vi "ReadHeadFast.vi"(9 "Use File?":bool=TRUE, 10 "raw reader":string, 11 "new file path":path=path "C:/WINDOWS/DESKTOP/rri.eye") -> (3 "refnum out":refnum<file>, 5 "Header In":T3={"header info"={"Header"="", "Head length"=0}, "A/D info"={"# rf points per line"=0, "# lines per scan"=0, "sample rate MHz"=0, "# A/D bits"=0, "# bytes per A/D"=0, "TGC Flag"=0, "A/D Type"=""}, "Tranducer Info"={"bandwidth"=0.0, "center freq"=0.0, "start freq"=0.0, "ID"=0}, "Scan Info"={"delay"=0.0, "pivot distance"=0.0, "sector scan angle"=0.0, "operator"="", "Scan Mode"="", "location"=""}, "Time/Date Info"={"date"="", "time"=""}, "RF Info"={"RF file name"="", "RF file att"="", "RF cal file name"="", "RF cal file att"=""}, "Patient Info"={"ID"="", "extended ID"="", "age"=0, "sex"="", "previously\nscanned"="", "PSA"=0.0, "LOS"=1, "Ethnicty 2"=3, "Race"=3}, "Tissue Type"={"organ"=0, "disease type"=0, "disease location"=0, "IQ_pts"=0, "RcvBuffer"=0, "RcvFrame"=0, "IQBuff"=0, "IQFrame"=0, "IQPage"=0}, "Votage scaling"={"Digitizer (dB)"=0.0, "Gain (dB)"=0.0, "Atten (dB)"=0.0}, "Comment"="", "Misc Info"={"avg num"=0, "c speed"=0, "Div By or SF zones"=0, "XMIT CHS"=0, "RCV CHS"=0, "Xmit angle"=0.0}, "Therapy Parameters"={"Theraputic Freq (MHz)"=0.1, "Time on (s)"=1.0, "Therapy amplitude (mV)"=50.0, "Lines Before"=20, "Lines After"=80}, "Scan Settings"={"Energy (uJ or V)"=0, "Damp (Ohm) or Fc"=0, "HP Filt (KHz)"=0, "LP Filt (MHz)"=0, "Gain (db)"=0, "prf (kHz)"=0.0, "Distance between\nscan lines (um)"=0, "Distance between\nscan planes (um)"=0, "Scan line gap (um)"=0.0, "Scan plane gap (um)"=0.0}, "Compression Parameters"={"F1 (MHz)"=0.0, "F2 (MHz)"=0.0, "% taper"=0.0, "duration"=0.0}, "Patient Info Xtra"={"First Name"="", "Last Name"="", "Notes"=""}, "ROI Box"=[]} {"Compression Parameters"."% taper" min=50 max=1000 format="%.2f"; "Compression Parameters"."F2 (MHz)" format="%.3f"; "Compression Parameters"."F1 (MHz)" format="%.3f"; "Scan Settings"."prf (kHz)" format="%.2f"; "Therapy Parameters"."Therapy amplitude (mV)" min=50 max=1000 format="%.2f"; "Therapy Parameters"."Time on (s)" format="%.3f"; "Therapy Parameters"."Theraputic Freq (MHz)" format="%.3f"; "Patient Info"."Race" items=["Am Ind or Alaska", "Asian", "Hawaiian, Pac Isl", "Black or Afr Amer", "White", "more than one race", "unknown"]; "Patient Info"."Ethnicty 2" items=["Hispanic", "Non-Hispanic", "unknown"]; "Patient Info"."LOS" items=["1", "2", "3", "4", "5"]; "Patient Info"."PSA" format="%.1f"; "Scan Info"."delay" format="%.2f"; "Scan Info"."pivot distance" format="%.2f"; "Scan Info"."sector scan angle" format="%.2f"; "Tranducer Info"."bandwidth" format="%.2f"; "Tranducer Info"."center freq" format="%.2f"; "Tranducer Info"."start freq" format="%.2f"}, 6 "Scan Settings (Pulser and Scaping)":T4 {"prf (kHz)" format="%.2f"}, 7 "raw header out":string)   [LabVIEW 2022 SP3]
uses:
  Header.ctl
panel:
  out "filler 3":string
  out "Blank":string
  out "Patient Info Old":T1={"ID"="", "Extended ID"="", "age"=0, "gender"="", "previously\nscanned"="", "PSA"=0.0, "LOS"=1, "Ethnicty 3"=3} {"Ethnicty 3" items=["Am Ind or Alaska", "Asian, Pac Islander", "Black, not Hispanic", "Hispanic", "White, not hispanic", "other, unknown"]; "LOS" items=["1", "2", "3", "4", "5"]; "PSA" format="%.1f"}
  out "blank":i16
  out "Non-5900 Scan Setting":T2={"Flag"=0, "Puls mode"=3, "Voltage [V]"=0, "Freq. [MHz]"=0, "Gain [dB]"=0, "not used"=0.0, "Distance between\nscan lines (mm)"=0, "Distance between\nscan planes (mm)"=0, "Scan line gap (um)"=0.0, "Scan plane gap (um)"=0.0} {"Puls mode" items=["Half cycle positive", "Half cycle negegative", "Full cycle positive", "Full cycle negative"]; "not used" format="%.2f"}
  out "Ethnicty":u8(ring)=3 items=["Am Ind or Alaska", "Asian, Pac Islander", "Black, not Hispanic", "Hispanic", "White, not hispanic", "other, unknown"]
  # "© 2001-2014\nRiverside Research Institute"
  # "Old style race indicator"
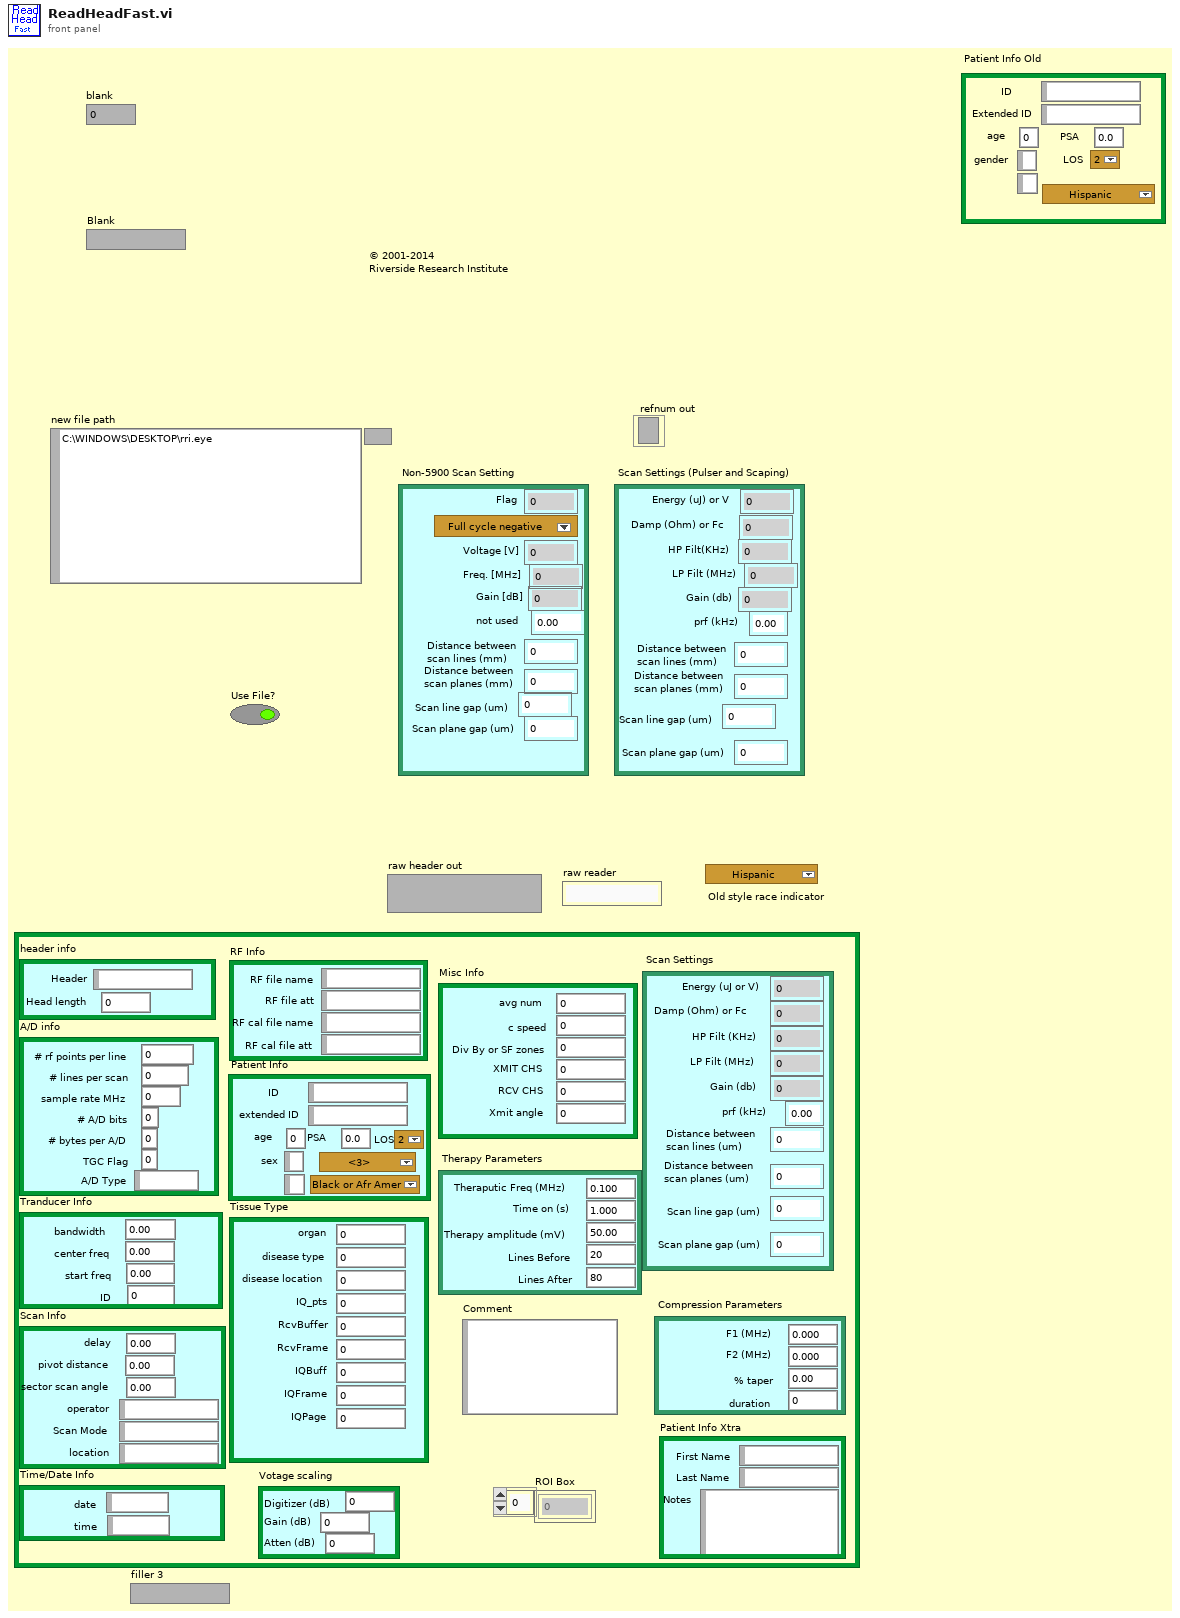
[diagram p1: front panel]
types:
  T1 = cluster{"ID":string, "Extended ID":string, "age":u16, "gender":string, "previously\nscanned":string, "PSA":sgl, "LOS":u8, "Ethnicty 3":u8}
  T2 = cluster{"Flag":u8, "Puls mode":u16, "Voltage [V]":u8, "Freq. [MHz]":u8, "Gain [dB]":u8, "not used":sgl, "Distance between\nscan lines (mm)":u16, "Distance between\nscan planes (mm)":u16, "Scan line gap (um)":sgl, "Scan plane gap (um)":sgl}
  T3 = typedef "Header.ctl" = cluster{"header info":cluster{"Header":string, "Head length":i16}, "A/D info":cluster{"# rf points per line":u16, "# lines per scan":u16, "sample rate MHz":u16, "# A/D bits":i16, "# bytes per A/D":u16, "TGC Flag":u16, "A/D Type":string}, "Tranducer Info":cluster{"bandwidth":sgl, "center freq":sgl, "start freq":sgl, "ID":i32}, "Scan Info":cluster{"delay":sgl, "pivot distance":sgl, "sector scan angle":sgl, "operator":string, "Scan Mode":string, "location":string}, "Time/Date Info":cluster{"date":string, "time":string}, "RF Info":cluster{"RF file name":string, "RF file att":string, "RF cal file name":string, "RF cal file att":string}, "Patient Info":cluster{"ID":string, "extended ID":string, "age":u16, "sex":string, "previously\nscanned":string, "PSA":sgl, "LOS":u8, "Ethnicty 2":u8, "Race":u8}, "Tissue Type":cluster{"organ":i16, "disease type":i16, "disease location":i16, "IQ_pts":u16, "RcvBuffer":u8, "RcvFrame":u16, "IQBuff":u8, "IQFrame":u16, "IQPage":u8}, "Votage scaling":cluster{"Digitizer (dB)":sgl, "Gain (dB)":sgl, "Atten (dB)":sgl}, "Comment":string, "Misc Info":cluster{"avg num":u16, "c speed":i16, "Div By or SF zones":i16, "XMIT CHS":u8, "RCV CHS":u8, "Xmit angle":sgl}, "Therapy Parameters":cluster{"Theraputic Freq (MHz)":sgl, "Time on (s)":sgl, "Therapy amplitude (mV)":sgl, "Lines Before":u16, "Lines After":u16}, "Scan Settings":cluster{"Energy (uJ or V)":u8, "Damp (Ohm) or Fc":u8, "HP Filt (KHz)":u8, "LP Filt (MHz)":u8, "Gain (db)":u8, "prf (kHz)":sgl, "Distance between\nscan lines (um)":u16, "Distance between\nscan planes (um)":u16, "Scan line gap (um)":sgl, "Scan plane gap (um)":sgl}, "Compression Parameters":cluster{"F1 (MHz)":sgl, "F2 (MHz)":sgl, "% taper":sgl, "duration":sgl}, "Patient Info Xtra":cluster{"First Name":string, "Last Name":string, "Notes":string}, "ROI Box":u16[]}
  T4 = cluster{"Energy (uJ) or V":u8, "Damp (Ohm) or Fc":u8, "HP Filt(KHz) ":u8, "LP Filt (MHz)":u8, "Gain (db)":u8, "prf (kHz)":sgl, "Distance between\nscan lines (mm)":u16, "Distance between\nscan planes (mm)":u16, "Scan line gap (um)":sgl, "Scan plane gap (um)":sgl}
  T5 = cluster{"Index":u16, "Index":u16, "Index":u16, "Index":u16, "Index":u16, "Index":u16, "raw reader":string}
  T6 = cluster{sgl, sgl, sgl, "raw reader":string, "raw reader":string, "raw reader":string}
  T7 = cluster{"raw reader":string, "raw reader":string}
  T8 = cluster{"raw reader":string, "raw reader":string, "raw reader":string, "raw reader":string}
  T9 = cluster{"raw reader":string, "raw reader":string, u16, "raw reader":string, "raw reader":string, sgl, i32, i32, i32}
  T10 = cluster{"raw reader":string, "raw reader":string, u16, "raw reader":string, "raw reader":string, sgl, i32, i32}
  T11 = cluster{"Index":i16, "Index":i16, "Index":i16, u16, "Index":u8, u16, "Index":u8, u16, "Index":u8}
  T12 = cluster{u16, "Index":i16, "Index":i16, "Index":u8, "Index":u8, sgl}
  T13 = cluster{u8, u8, u8, u8, u8, sgl, u16, u16, sgl, sgl}
  T14 = cluster{"raw reader":string, "raw reader":string, "raw reader":string}
  T15 = cluster{cluster{"raw reader":string, i16}, cluster{"Index":u16, "Index":u16, "Index":u16, "Index":u16, "Index":u16, "Index":u16, "raw reader":string}, cluster{sgl, sgl, sgl, i32}, cluster{sgl, sgl, sgl, "raw reader":string, "raw reader":string, "raw reader":string}, cluster{"raw reader":string, "raw reader":string}, cluster{"raw reader":string, "raw reader":string, "raw reader":string, "raw reader":string}, cluster{"raw reader":string, "raw reader":string, u16, "raw reader":string, "raw reader":string, sgl, i32, i32, i32}, cluster{"Index":i16, "Index":i16, "Index":i16, u16, "Index":u8, u16, "Index":u8, u16, "Index":u8}, cluster{sgl, sgl, sgl}, "raw reader":string, cluster{u16, "Index":i16, "Index":i16, "Index":u8, "Index":u8, sgl}, cluster{sgl, sgl, sgl, u16, u16}, cluster{u8, u8, u8, u8, u8, sgl, u16, u16, sgl, sgl}, cluster{sgl, sgl, sgl, sgl}, cluster{"raw reader":string, "raw reader":string, "raw reader":string}, u16[]}
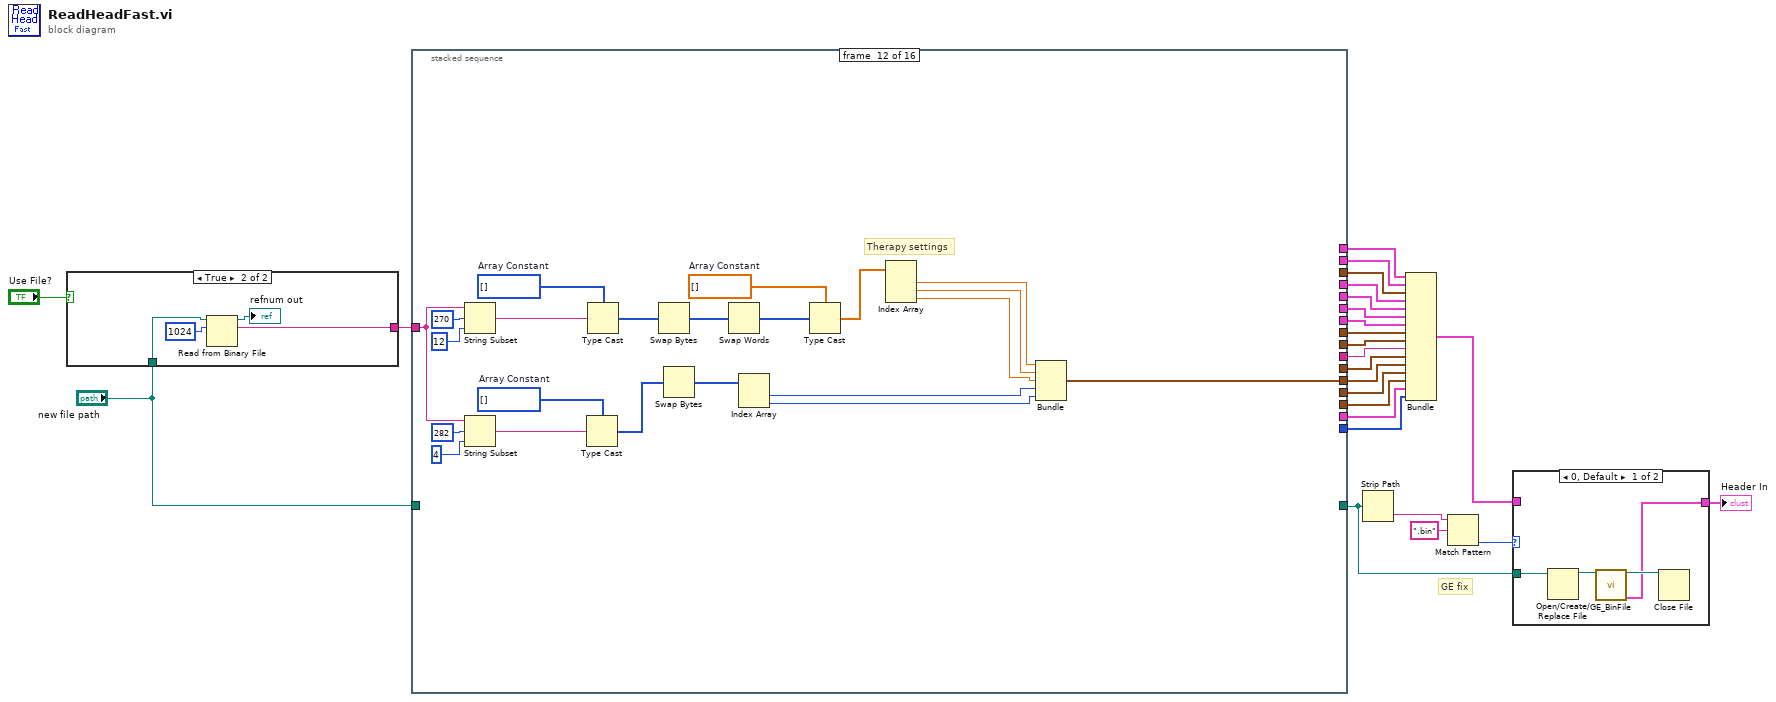
[diagram p0: block diagram]
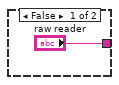
[diagram p3: hidden frame]
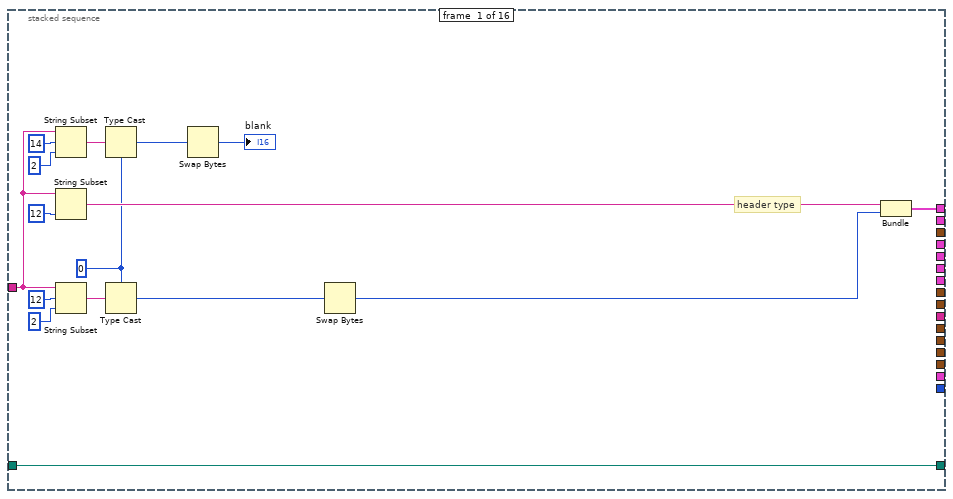
[diagram p4: hidden frame]
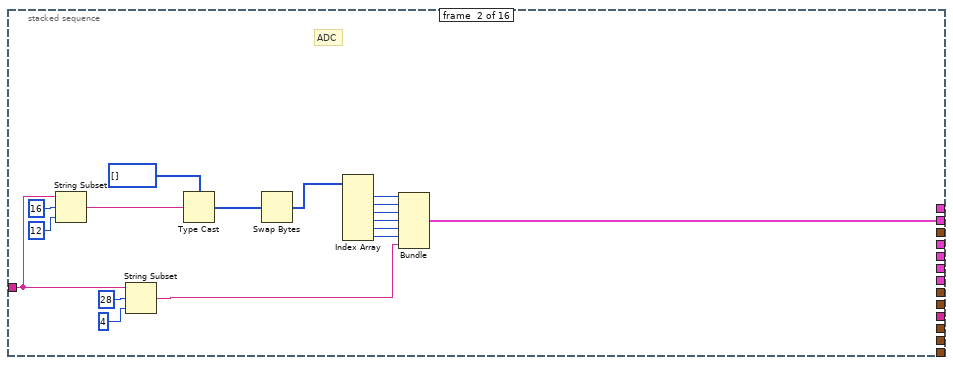
[diagram p5: hidden frame]
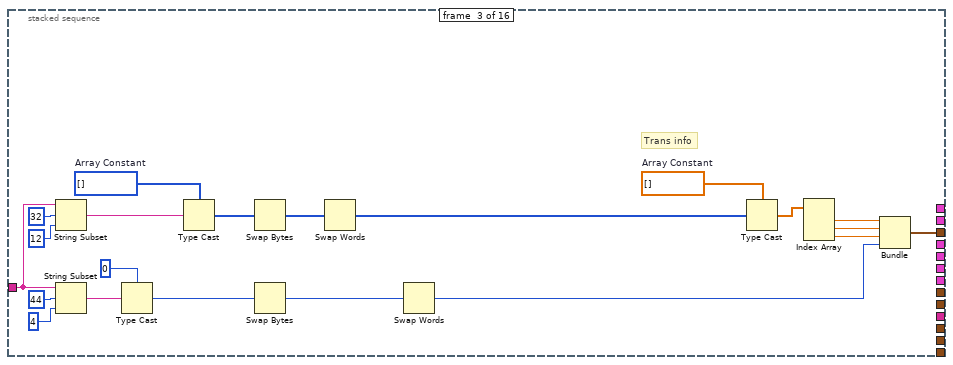
[diagram p6: hidden frame]
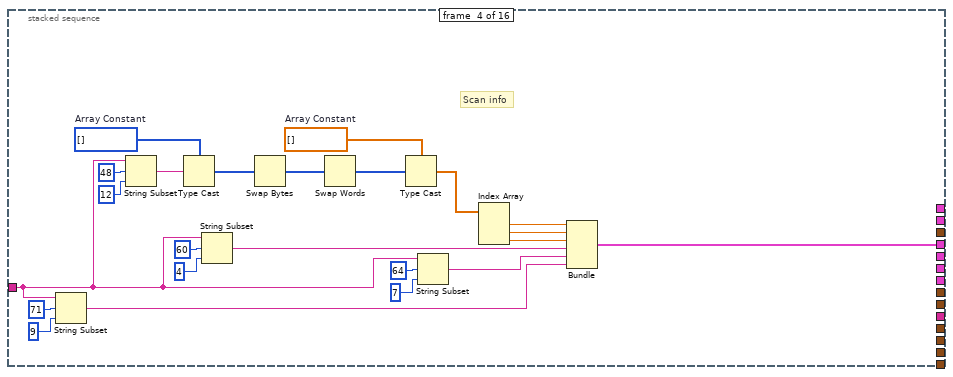
[diagram p7: hidden frame]
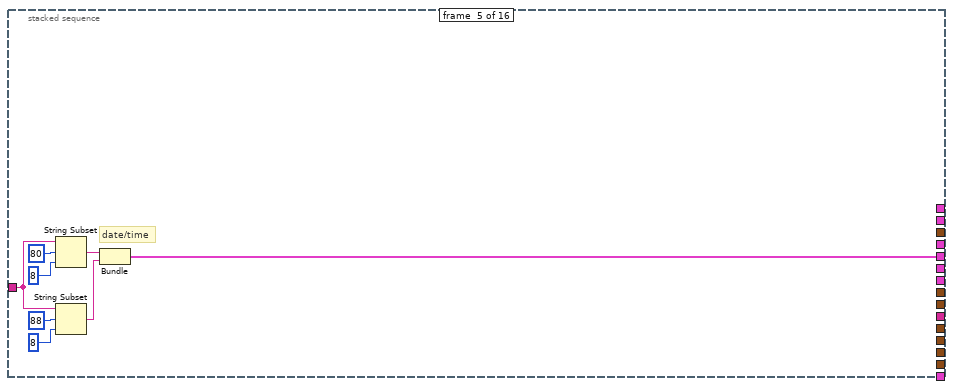
[diagram p8: hidden frame]
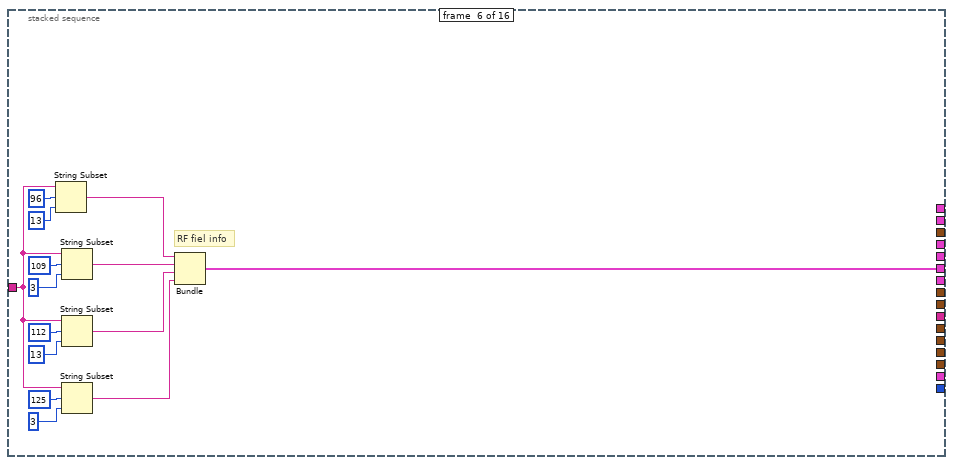
[diagram p9: hidden frame]
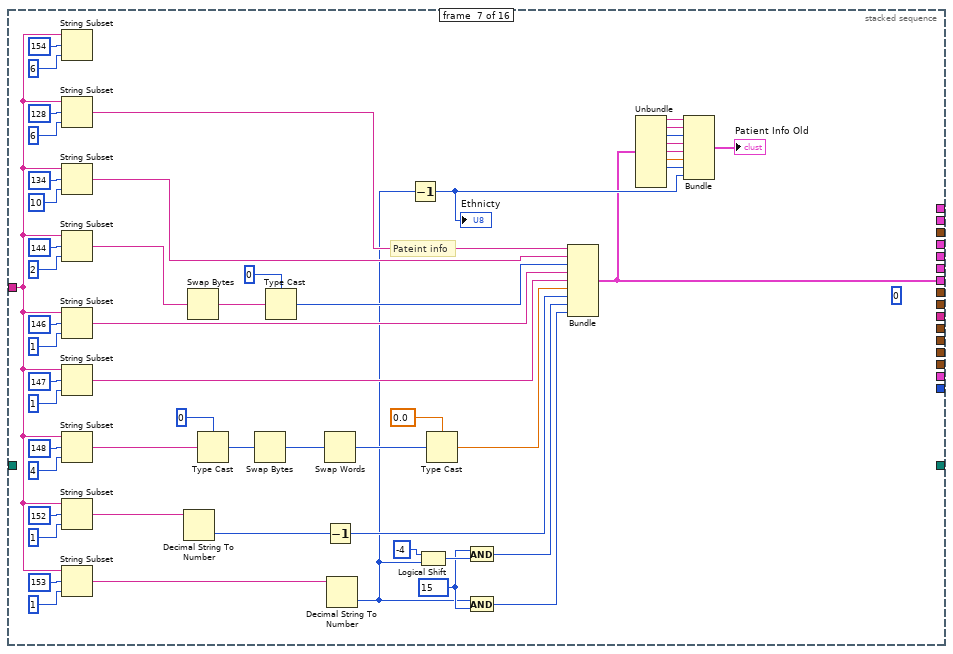
[diagram p10: hidden frame]
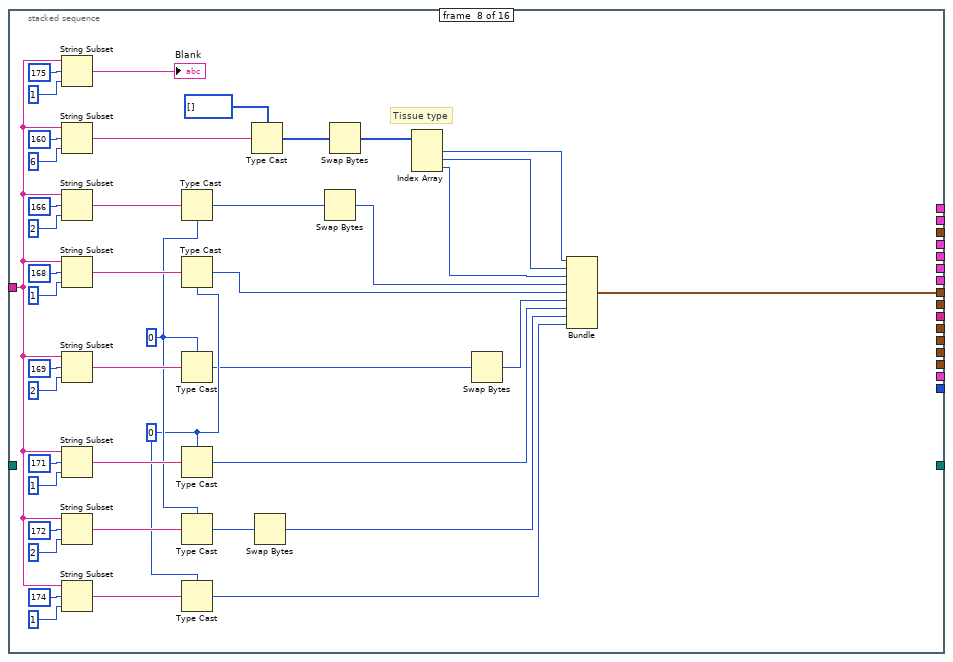
[diagram p11: hidden frame]
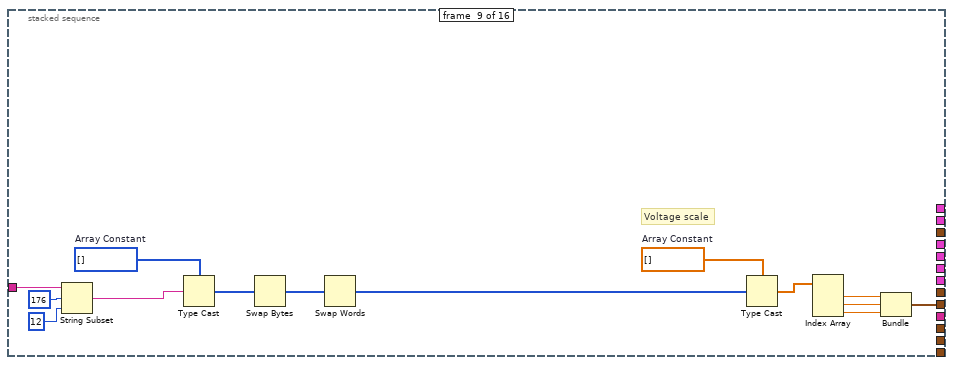
[diagram p12: hidden frame]
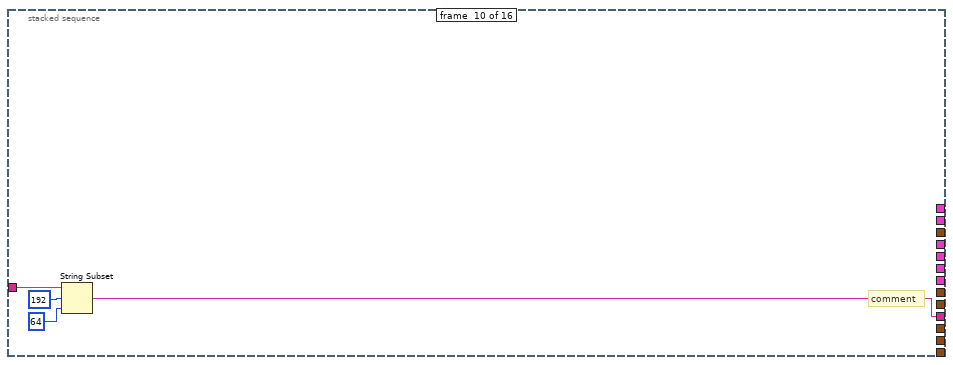
[diagram p13: hidden frame]
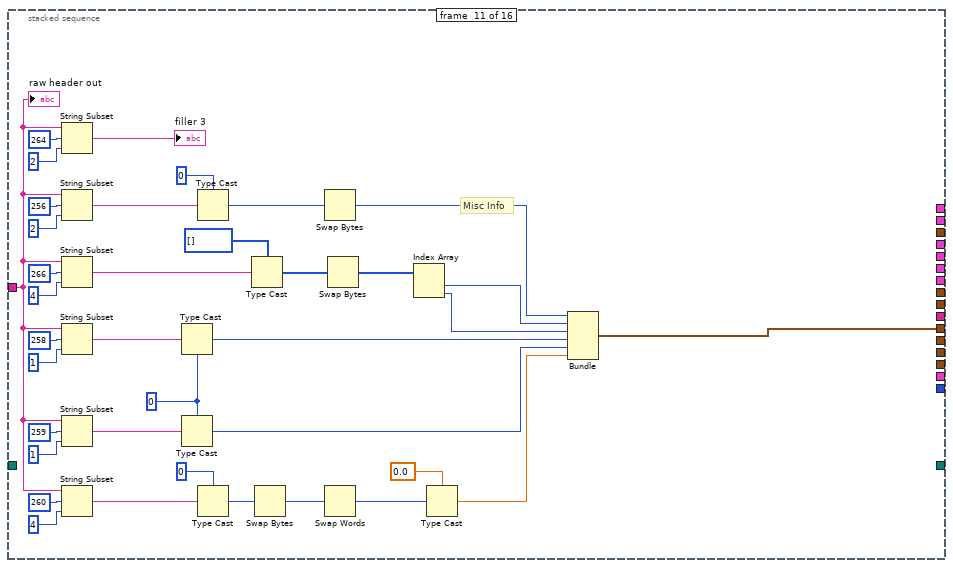
[diagram p14: hidden frame]
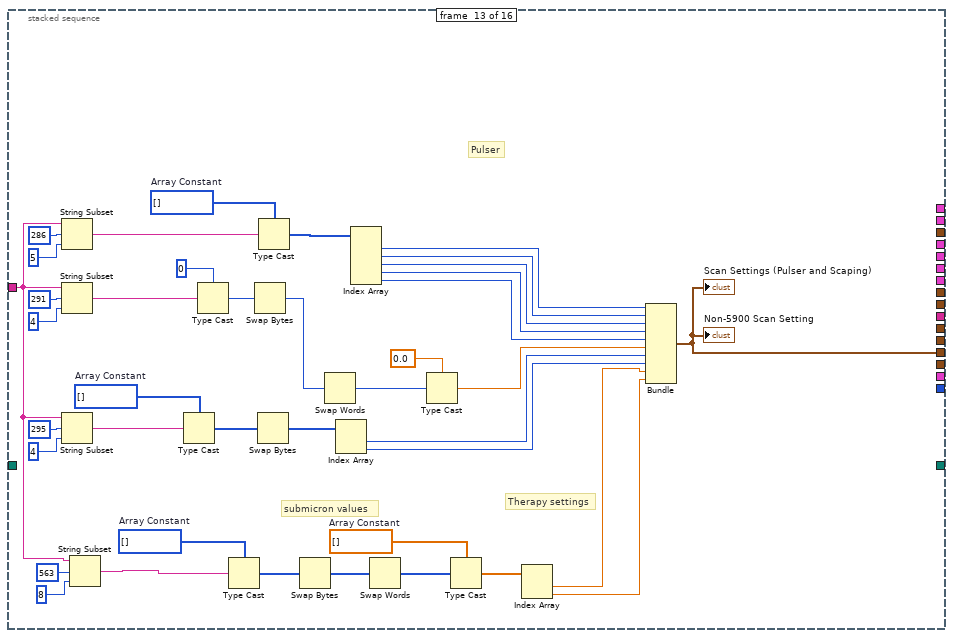
[diagram p15: hidden frame]
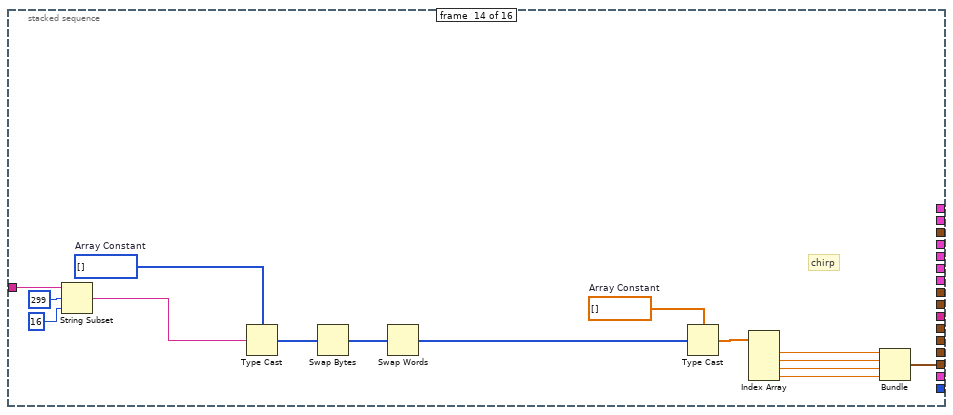
[diagram p16: hidden frame]
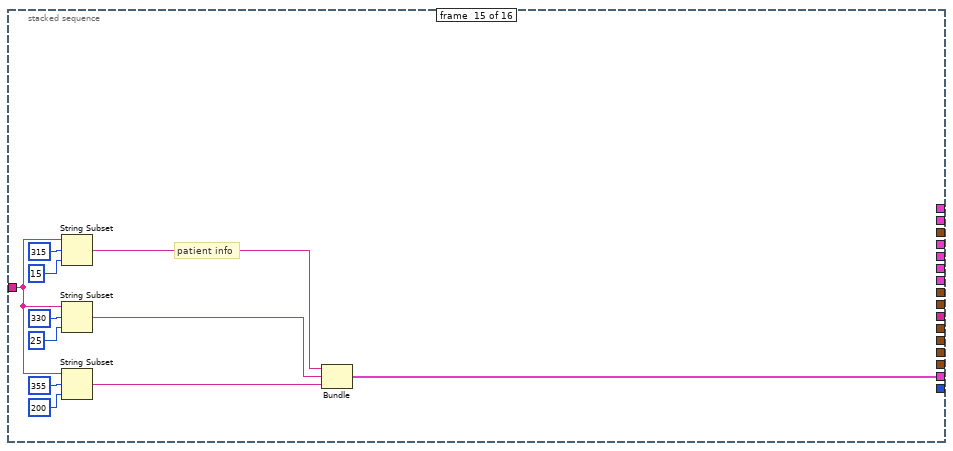
[diagram p17: hidden frame]
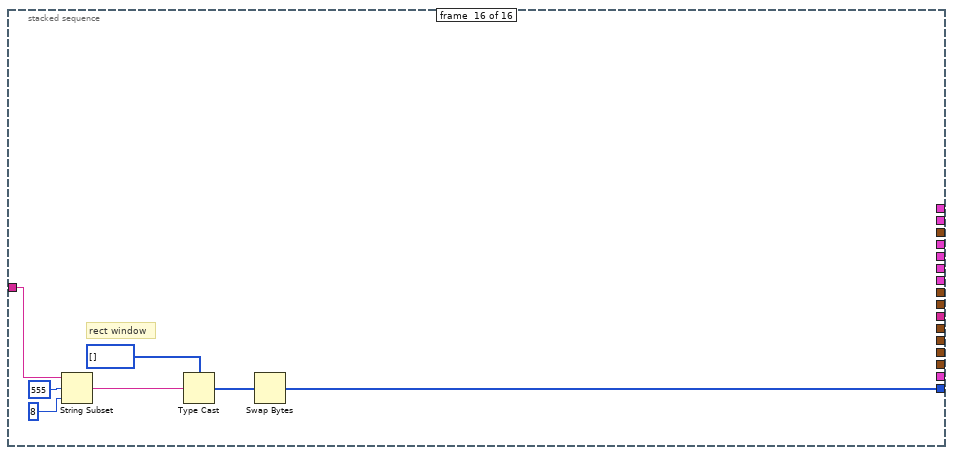
[diagram p18: hidden frame]
diagram:
  # "GE fix"
  n1 = case shown="True" "Use File?" {
    tunnel: ["raw reader" w29] -> w19
    tunnel: "new file path" -> [_ w27]
    frame False {
    }
    frame True {
      n2 = Read from Binary File(10:1024, 11:w27) -> (2:w29:string, 3:→"refnum out":refnum<file>)  [unwired: 1 in, 5 out]
    }
  }
  n3 = stacked-sequence {
    tunnel: [w41 _ _ _ _ _ _ _ _ _ _ _ _ _ _ _] -> w25
    tunnel: [_ _ _ w103 _ _ _ _ _ _ _ _ _ _ _ _] -> w24
    tunnel: [_ _ _ _ w113 _ _ _ _ _ _ _ _ _ _ _] -> w23
    tunnel: [_ _ _ _ _ _ _ _ _ w244 _ _ _ _ _ _] -> w22
    tunnel: [_ _ _ _ _ w125 _ _ _ _ _ _ _ _ _ _] -> w21
    tunnel: w19 -> [w45 w60 w82 w102 w109 w116 w164 w204 w234 w241 w247 w301 w319 w355 w360 w374]
    tunnel: [_ _ _ _ _ _ _ _ _ _ _ _ _ w357 _ _] -> w20
    tunnel: [_ w58 _ _ _ _ _ _ _ _ _ _ _ _ _ _] -> w18
    tunnel: [_ _ w80 _ _ _ _ _ _ _ _ _ _ _ _ _] -> w17
    tunnel: [_ _ _ _ _ _ w138 _ _ _ _ _ _ _ _ _] -> w16
    tunnel: [_ _ _ _ _ _ _ w220 _ _ _ _ _ _ _ _] -> w15
    tunnel: [_ _ _ _ _ _ _ _ w229 _ _ _ _ _ _ _] -> w14
    tunnel: [_ _ _ _ _ _ _ _ _ _ w279 _ _ _ _ _] -> w13
    tunnel: [_ _ _ _ _ _ _ _ _ _ _ w295 _ _ _ _] -> w12
    tunnel: [_ _ _ _ _ _ _ _ _ _ _ _ w331 _ _ _] -> w11
    tunnel: [_ _ _ _ _ _ _ _ _ _ _ _ _ _ w359 _] -> w9
    tunnel: [_ _ _ _ _ _ _ _ _ _ _ _ _ _ _ w370] -> w8
    tunnel: [w31 _ _ _ _ _ _ _ _ _ _ _ _ _ _ _] -> w3
    tunnel: "new file path" -> [w31 _ _ _ _ _ _ _ _ _ _ _ _ _ _ _]
    frame #0 {
      w42 = i16 0 ("Index")
      # "header type"
      n4 = String Subset(string=w45, offset (0)=14 ("count"), length (rest)=2) -> (substring=w34:string)
      n5 = String Subset(string=w45, length (rest)=12 ("count")) -> (substring=w46:string)  [unwired: 1 out]
      n6 = String Subset(string=w45, offset (0)=12 ("count"), length (rest)=2) -> (substring=w37:string)
      n7 = Type Cast(type=w42, x=w34) -> (*(type *) &x=w33:i16)
      n8 = Type Cast(type=w42, x=w37) -> (*(type *) &x=w36:i16)
      n9 = Swap Bytes(anything=w33) -> (byte swapped=→"blank":i16)
      n10 = Swap Bytes(anything=w36) -> (byte swapped=w35:i16)
      n11 = Bundle("raw reader"=w46, w35) -> (w41:cluster{"raw reader":string, i16})  [unwired: 1 out]
    }
    frame #1 {
      # "ADC"
      n12 = String Subset(string=w60, offset (0)=16 ("pos offset (0)"), length (rest)=12 ("count")) -> (substring=w54:string)
      n13 = String Subset(string=w60, offset (0)=28, length (rest)=4 ("count")) -> (substring=w62:string)
      n14 = Type Cast(type=u16[] [], x=w54) -> (*(type *) &x=w53:u16[])
      n15 = Swap Bytes(anything=w53) -> (byte swapped=w52:u16[])
      n16 = Index Array(array=w52) -> (element #1=w63:u16, element #2=w51:u16, element #3=w50:u16, element #4=w49:u16, element #5=w48:u16, element #6=w47:u16)  [unwired: 6 in]
      n17 = Bundle("Index"=w63, "Index"=w51, "Index"=w50, "Index"=w49, "Index"=w48, "Index"=w47, "raw reader"=w62) -> (w58:T5)  [unwired: 1 out]
    }
    frame #2 {
      w68 = sgl[] []  # Array Constant
      w84 = i32[] []  # Array Constant
      # "Trans info"
      n18 = String Subset(string=w82, offset (0)=32 ("pos offset (0)"), length (rest)=12 ("count")) -> (substring=w75:string)
      n19 = String Subset(string=w82, offset (0)=44 ("count"), length (rest)=4 ("byte stream type")) -> (substring=w69:string)
      n20 = Type Cast(type=0, x=w69) -> (*(type *) &x=w70:i32)
      n21 = Type Cast(type=w84, x=w75) -> (*(type *) &x=w73:i32[])
      n22 = Swap Bytes(anything=w73) -> (byte swapped=w74:i32[])
      n23 = Swap Bytes(anything=w70) -> (byte swapped=w72:i32)
      n24 = Swap Words(1:w74) -> (0:w67:i32[])
      n25 = Swap Words(1:w72) -> (0:w71:i32)
      n26 = Type Cast(type=w68, x=w67) -> (*(type *) &x=w66:sgl[])
      n27 = Index Array(array=w66) -> (element #1=w83:sgl, element #2=w65:sgl, element #3=w64:sgl)  [unwired: 3 in]
      n28 = Bundle(w83, w65, w64, w71) -> (w80:cluster{sgl, sgl, sgl, i32})  [unwired: 1 out]
    }
    frame #3 {
      w87 = i32[] []  # Array Constant
      w88 = sgl[] []  # Array Constant
      # "Scan info"
      n29 = String Subset(string=w102, offset (0)=71 ("pos offset (0)"), length (rest)=9 ("count")) -> (substring=w104:string)
      n30 = String Subset(string=w102, offset (0)=48 ("pos offset (0)"), length (rest)=12 ("count")) -> (substring=w94:string)
      n31 = Type Cast(type=w87, x=w94) -> (*(type *) &x=w92:i32[])
      n32 = String Subset(string=w102, offset (0)=60 ("pos offset (0)"), length (rest)=4 ("count")) -> (substring=w106:string)
      n33 = Swap Bytes(anything=w92) -> (byte swapped=w93:i32[])
      n34 = Swap Words(1:w93) -> (0:w90:i32[])
      n35 = Type Cast(type=w88, x=w90) -> (*(type *) &x=w89:sgl[])
      n36 = String Subset(string=w102, offset (0)=64 ("pos offset (0)"), length (rest)=7 ("count")) -> (substring=w105:string)
      n37 = Index Array(array=w89) -> (element #1=w107:sgl, element #2=w86:sgl, element #3=w85:sgl)  [unwired: 3 in]
      n38 = Bundle(w107, w86, w85, "raw reader"=w106, "raw reader"=w105, "raw reader"=w104) -> (w103:T6)  [unwired: 1 out]
    }
    frame #4 {
      # "date/time"
      n39 = String Subset(string=w109, offset (0)=80 ("pos offset (0)"), length (rest)=8 ("count")) -> (substring=w115:string)
      n40 = String Subset(string=w109, offset (0)=88, length (rest)=8 ("count")) -> (substring=w114:string)
      n41 = Bundle("raw reader"=w115, "raw reader"=w114) -> (w113:T7)  [unwired: 1 out]
    }
    frame #5 {
      # "RF fiel info"
      n42 = String Subset(string=w116, offset (0)=96 ("pos offset (0)"), length (rest)=13 ("count")) -> (substring=w129:string)
      n43 = String Subset(string=w116, offset (0)=109, length (rest)=3 ("count")) -> (substring=w128:string)
      n44 = String Subset(string=w116, offset (0)=112, length (rest)=13 ("count")) -> (substring=w127:string)
      n45 = String Subset(string=w116, offset (0)=125, length (rest)=3 ("count")) -> (substring=w126:string)
      n46 = Bundle("raw reader"=w129, "raw reader"=w128, "raw reader"=w127, "raw reader"=w126) -> (w125:T8)  [unwired: 1 out]
    }
    frame #6 {
      w175 = 15
      (unwired) u16 0
      # "Pateint info"
      n47 = String Subset(string=w164, offset (0)=154, length (rest)=6 ("count")) -> ()  [unwired: 1 out]
      n48 = String Subset(string=w164, offset (0)=128 ("pos offset (0)"), length (rest)=6 ("count")) -> (substring=w182:string)
      n49 = String Subset(string=w164, offset (0)=134, length (rest)=10 ("count")) -> (substring=w181:string)
      n50 = String Subset(string=w164, offset (0)=144, length (rest)=2 ("count")) -> (substring=w183:string)
      n51 = String Subset(string=w164, offset (0)=146, length (rest)=1 ("count")) -> (substring=w180:string)
      n52 = String Subset(string=w164, offset (0)=147, length (rest)=1 ("count")) -> (substring=w179:string)
      n53 = String Subset(string=w164, offset (0)=148, length (rest)=4 ("count")) -> (substring=w134:string)
      n54 = String Subset(string=w164, offset (0)=152, length (rest)=1 ("count")) -> (substring=w141:string)
      n55 = String Subset(string=w164, offset (0)=153, length (rest)=1 ("count")) -> (substring=w139:string)
      n56 = Decimal String To Number(string=w141) -> (number=w140:i32)  [unwired: 3 out]
      n57 = Swap Bytes(anything=w183) -> (byte swapped=w145:string)
      n58 = Type Cast(type=0, x=w134) -> (*(type *) &x=w136:i32)
      n59 = Swap Bytes(anything=w136) -> (byte swapped=w135:i32)
      n60 = Type Cast(type=u16 0, x=w145) -> (*(type *) &x=w144:u16)
      n61 = Swap Words(1:w135) -> (0:w137:i32)
      n62 = Decrement(x=w140) -> (x-1=w178:i32)
      n63 = Decimal String To Number(string=w139) -> (number=w130:i32)  [unwired: 3 out]
      n64 = Decrement(x=w130) -> (x-1=w165:i32)
      "Ethnicty" <- w165
      n65 = Logical Shift(y=-4, x=w130) -> (x << y=w176:i32)
      n66 = Type Cast(type=sgl 0.0, x=w137) -> (*(type *) &x=w133:sgl)
      n67 = And(x=w175, y=w176) -> (x .and. y?=w174:i32)
      n68 = And(x=w130, y=w175) -> (x .and. y?=w173:i32)
      n69 = Bundle("raw reader"=w182, "raw reader"=w181, w144, "raw reader"=w180, "raw reader"=w179, w133, w178, w174, w173) -> (w138:T9)  [unwired: 1 out]
      n70 = Unbundle(w138) -> ("raw reader"=w172:string, "raw reader"=w171:string, w170:u16, "raw reader"=w169:string, "raw reader"=w168:string, w167:sgl, w166:i32)  [unwired: 2 out]
      n71 = Bundle("raw reader"=w172, "raw reader"=w171, w170, "raw reader"=w169, "raw reader"=w168, w167, w166, w165) -> (→"Patient Info Old":T10)  [unwired: 1 out]
    }
    frame #7 {
      w196 = u8 0 ("Index")
      w197 = u16 0 ("Index")
      # "Tissue type"
      n72 = String Subset(string=w204, offset (0)=175, length (rest)=1 ("count")) -> (substring=→"Blank":string)
      n73 = String Subset(string=w204, offset (0)=160 ("pos offset (0)"), length (rest)=6 ("count")) -> (substring=w217:string)
      n74 = String Subset(string=w204, offset (0)=166 ("pos offset (0)"), length (rest)=2 ("count")) -> (substring=w203:string)
      n75 = String Subset(string=w204, offset (0)=168 ("pos offset (0)"), length (rest)=1 ("count")) -> (substring=w202:string)
      n76 = String Subset(string=w204, offset (0)=169 ("pos offset (0)"), length (rest)=2 ("count")) -> (substring=w201:string)
      n77 = String Subset(string=w204, offset (0)=171 ("pos offset (0)"), length (rest)=1 ("count")) -> (substring=w198:string)
      n78 = String Subset(string=w204, offset (0)=172 ("pos offset (0)"), length (rest)=2 ("count")) -> (substring=w200:string)
      n79 = String Subset(string=w204, offset (0)=174 ("pos offset (0)"), length (rest)=1 ("count")) -> (substring=w199:string)
      n80 = Type Cast(type=w197, x=w203) -> (*(type *) &x=w187:u16)
      n81 = Type Cast(type=w196, x=w202) -> (*(type *) &x=w195:u8)
      n82 = Type Cast(type=w197, x=w201) -> (*(type *) &x=w189:u16)
      n83 = Type Cast(type=w196, x=w198) -> (*(type *) &x=w194:u8)
      n84 = Type Cast(type=w197, x=w200) -> (*(type *) &x=w191:u16)
      n85 = Type Cast(type=w196, x=w199) -> (*(type *) &x=w193:u8)
      n86 = Type Cast(type=i16[] [], x=w217) -> (*(type *) &x=w219:i16[])
      n87 = Swap Bytes(anything=w191) -> (byte swapped=w190:u16)
      n88 = Swap Bytes(anything=w187) -> (byte swapped=w186:u16)
      n89 = Swap Bytes(anything=w219) -> (byte swapped=w218:i16[])
      n90 = Index Array(array=w218) -> (element #1=w226:i16, element #2=w185:i16, element #3=w184:i16)  [unwired: 3 in]
      n91 = Swap Bytes(anything=w189) -> (byte swapped=w188:u16)
      n92 = Bundle("Index"=w226, "Index"=w185, "Index"=w184, w186, "Index"=w195, w188, "Index"=w194, w190, "Index"=w193) -> (w220:T11)  [unwired: 1 out]
    }
    frame #8 {
      w236 = i32[] []  # Array Constant
      w237 = sgl[] []  # Array Constant
      # "Voltage scale"
      n93 = String Subset(string=w234, offset (0)=176 ("pos offset (0)"), length (rest)=12 ("pos offset (0)")) -> (substring=w235:string)
      n94 = Type Cast(type=w236, x=w235) -> (*(type *) &x=w239:i32[])
      n95 = Swap Bytes(anything=w239) -> (byte swapped=w240:i32[])
      n96 = Swap Words(1:w240) -> (0:w238:i32[])
      n97 = Type Cast(type=w237, x=w238) -> (*(type *) &x=w231:sgl[])
      n98 = Index Array(array=w231) -> (element #1=w230:sgl, element #2=w227:sgl, element #3=w228:sgl)  [unwired: 3 in]
      n99 = Bundle(w230, w227, w228) -> (w229:cluster{sgl, sgl, sgl})  [unwired: 1 out]
    }
    frame #9 {
      # "comment"
      n100 = String Subset(string=w241, offset (0)=192 ("pos offset (0)"), length (rest)=64 ("count")) -> (substring=w244:string)
    }
    frame #10 {
      w260 = u8 0 ("Index")
      # "Misc Info"
      n101 = String Subset(string=w247, offset (0)=264, length (rest)=2 ("count")) -> (substring=→"filler 3":string)
      n102 = String Subset(string=w247, offset (0)=256 ("pos offset (0)"), length (rest)=2 ("count")) -> (substring=w271:string)
      n103 = String Subset(string=w247, offset (0)=266, length (rest)=4 ("count")) -> (substring=w269:string)
      n104 = String Subset(string=w247, offset (0)=258 ("pos offset (0)"), length (rest)=1 ("count")) -> (substring=w264:string)
      n105 = String Subset(string=w247, offset (0)=259 ("pos offset (0)"), length (rest)=1 ("count")) -> (substring=w261:string)
      n106 = String Subset(string=w247, offset (0)=260, length (rest)=4 ("count")) -> (substring=w250:string)
      n107 = Type Cast(type=w260, x=w264) -> (*(type *) &x=w258:u8)
      n108 = Type Cast(type=w260, x=w261) -> (*(type *) &x=w257:u8)
      n109 = Type Cast(type=u16 0 ("Index"), x=w271) -> (*(type *) &x=w270:u16)
      n110 = Type Cast(type=0, x=w250) -> (*(type *) &x=w254:i32)
      n111 = Type Cast(type=i16[] [], x=w269) -> (*(type *) &x=w268:i16[])
      n112 = Swap Bytes(anything=w254) -> (byte swapped=w253:i32)
      n113 = Swap Bytes(anything=w270) -> (byte swapped=w259:u16)
      n114 = Swap Words(1:w253) -> (0:w255:i32)
      n115 = Swap Bytes(anything=w268) -> (byte swapped=w267:i16[])
      n116 = Index Array(array=w267) -> (element #1=w281:i16, element #2=w245:i16)  [unwired: 2 in]
      n117 = Type Cast(type=sgl 0.0, x=w255) -> (*(type *) &x=w246:sgl)
      n118 = Bundle(w259, "Index"=w281, "Index"=w245, "Index"=w258, "Index"=w257, w246) -> (w279:T12)  [unwired: 1 out]
      "raw header out" <- w247
    }
    frame #11 {
      w287 = i32[] []  # Array Constant
      w288 = sgl[] []  # Array Constant
      w296 = u16[] []  # Array Constant
      # "Therapy settings"
      n119 = String Subset(string=w301, offset (0)=270 ("pos offset (0)"), length (rest)=12 ("count")) -> (substring=w286:string)
      n120 = String Subset(string=w301, offset (0)=282 ("count"), length (rest)=4) -> (substring=w292:string)
      n121 = Type Cast(type=w296, x=w292) -> (*(type *) &x=w294:u16[])
      n122 = Type Cast(type=w287, x=w286) -> (*(type *) &x=w290:i32[])
      n123 = Swap Bytes(anything=w290) -> (byte swapped=w291:i32[])
      n124 = Swap Bytes(anything=w294) -> (byte swapped=w293:u16[])
      n125 = Swap Words(1:w291) -> (0:w289:i32[])
      n126 = Index Array(array=w293) -> (element #1=w302:u16, element #2=w282:u16)  [unwired: 2 in]
      n127 = Type Cast(type=w288, x=w289) -> (*(type *) &x=w285:sgl[])
      n128 = Index Array(array=w285) -> (element #1=w303:sgl, element #2=w284:sgl, element #3=w283:sgl)  [unwired: 3 in]
      n129 = Bundle(w303, w284, w283, w302, w282) -> (w295:cluster{sgl, sgl, sgl, u16, u16})  [unwired: 1 out]
    }
    frame #12 {
      w314 = i32[] []  # Array Constant
      w315 = sgl[] []  # Array Constant
      w333 = u16[] []  # Array Constant
      w339 = u8[] []  # Array Constant
      # "submicron values"
      # "Therapy settings"
      # "Pulser"
      n130 = String Subset(string=w319, offset (0)=286 ("pos offset (0)"), length (rest)=5 ("count")) -> (substring=w341:string)
      n131 = String Subset(string=w319, offset (0)=291, length (rest)=4 ("count")) -> (substring=w322:string)
      n132 = String Subset(string=w319, offset (0)=295, length (rest)=4 ("count")) -> (substring=w330:string)
      n133 = String Subset(string=w319, offset (0)=563, length (rest)=8 ("count")) -> (substring=w312:string)
      n134 = Type Cast(type=w333, x=w330) -> (*(type *) &x=w329:u16[])
      n135 = Type Cast(type=0, x=w322) -> (*(type *) &x=w326:i32)
      n136 = Type Cast(type=w314, x=w312) -> (*(type *) &x=w317:i32[])
      n137 = Swap Bytes(anything=w326) -> (byte swapped=w327:i32)
      n138 = Swap Bytes(anything=w329) -> (byte swapped=w328:u16[])
      n139 = Type Cast(type=w339, x=w341) -> (*(type *) &x=w340:u8[])
      n140 = Swap Bytes(anything=w317) -> (byte swapped=w318:i32[])
      n141 = Swap Words(1:w327) -> (0:w325:i32)
      n142 = Index Array(array=w328) -> (element #1=w343:u16, element #2=w304:u16)  [unwired: 2 in]
      n143 = Index Array(array=w340) -> (element #1=w332:u8, element #2=w308:u8, element #3=w307:u8, element #4=w306:u8, element #5=w305:u8)  [unwired: 5 in]
      n144 = Swap Words(1:w318) -> (0:w316:i32[])
      n145 = Type Cast(type=sgl 0.0, x=w325) -> (*(type *) &x=w324:sgl)
      n146 = Type Cast(type=w315, x=w316) -> (*(type *) &x=w313:sgl[])
      n147 = Index Array(array=w313) -> (element #1=w310:sgl, element #2=w309:sgl)  [unwired: 2 in]
      n148 = Bundle(w332, w308, w307, w306, w305, w324, w343, w304, w310, w309) -> (w331:T13)  [unwired: 1 out]
      "Scan Settings (Pulser and Scaping)" <- w331
      "Non-5900 Scan Setting" <- w331
    }
    frame #13 {
      w349 = i32[] []  # Array Constant
      w350 = sgl[] []  # Array Constant
      # "chirp"
      n149 = String Subset(string=w355, offset (0)=299 ("pos offset (0)"), length (rest)=16 ("count")) -> (substring=w348:string)
      n150 = Type Cast(type=w349, x=w348) -> (*(type *) &x=w352:i32[])
      n151 = Swap Bytes(anything=w352) -> (byte swapped=w353:i32[])
      n152 = Swap Words(1:w353) -> (0:w351:i32[])
      n153 = Type Cast(type=w350, x=w351) -> (*(type *) &x=w347:sgl[])
      n154 = Index Array(array=w347) -> (element #1=w358:sgl, element #2=w346:sgl, element #3=w345:sgl, element #4=w344:sgl)  [unwired: 4 in]
      n155 = Bundle(w358, w346, w345, w344) -> (w357:cluster{sgl, sgl, sgl, sgl})  [unwired: 1 out]
    }
    frame #14 {
      # "patient info"
      n156 = String Subset(string=w360, offset (0)=315 ("pos offset (0)"), length (rest)=15 ("count")) -> (substring=w363:string)
      n157 = String Subset(string=w360, offset (0)=330 ("pos offset (0)"), length (rest)=25 ("count")) -> (substring=w362:string)
      n158 = String Subset(string=w360, offset (0)=355 ("pos offset (0)"), length (rest)=200 ("count")) -> (substring=w361:string)
      n159 = Bundle("raw reader"=w363, "raw reader"=w362, "raw reader"=w361) -> (w359:T14)  [unwired: 1 in]
    }
    frame #15 {
      # "rect window"
      n160 = String Subset(string=w374, offset (0)=555 ("pos offset (0)"), length (rest)=8 ("count")) -> (substring=w373:string)
      n161 = Type Cast(type=u16[] [], x=w373) -> (*(type *) &x=w371:u16[])
      n162 = Swap Bytes(anything=w371) -> (byte swapped=w370:u16[])
    }
  }
  n163 = Strip Path(path=w3) -> (name=w6:string)  [unwired: 1 out]
  n164 = Bundle(w25, w18, w17, w24, w23, w21, w16, w15, w14, "raw reader"=w22, w13, w12, w11, w20, w9, w8) -> (w4:T15)  [unwired: 1 out]
  n165 = Match Pattern(string=w6, regular expression=".bin") -> (offset past match=w5:i32)  [unwired: 1 in, 3 out]
  n166 = case shown="0, Default" w5 {
    tunnel: w4 -> [_ w381]
    tunnel: w3 -> [w380 _]
    tunnel: [w377 w381] -> w2
    frame 0, Default {
      n167 = Open/Create/Replace File(file path (use dialog)=w380) -> (refnum out=w379:refnum<file>)  [unwired: 5 in, 2 out]
      n168 = call "GE_BinFile.vi"("refnum"=w379) -> ("refnum out"=w378:refnum<file>, "Header In"=w377:T3)  [unwired: 9 in, 4 out]
      n169 = Close File(refnum=w378) -> ()  [unwired: 1 in, 2 out]
    }
    frame -1 {
    }
  }
  "Header In" <- w2
